vi "Test One Line State String Unwired.vi"(8 "error in (no error)":errorcluster) -> (0 "error out":errorcluster)   [LabVIEW 2013, in "JKI State Machine API - Tests.lvlib"]
uses:
  JKI State Machine API - Tests.lvlib
  source/JKI State Machine API.lvlib
  <vilib>/addons/_JKI Toolkits/Caraya/classes/Test/Test.lvclass
  <vilib>/addons/_JKI Toolkits/Caraya/classes/Assert/Assert.lvclass
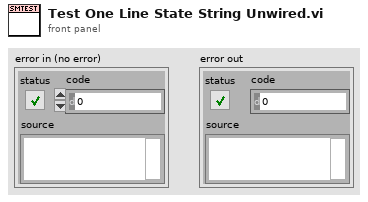
[diagram p1: front panel]
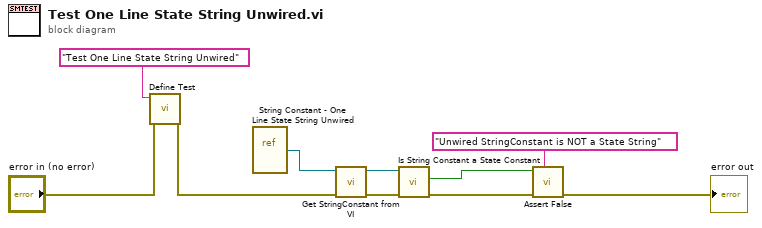
[diagram p0: block diagram]
diagram:
  n1 = call <vilib>:"Define Test.vi"("error in (no error)"="error in (no error)", "Label (VI Title)"="Test One Line State String Unwired") -> ("error out"=w9:errorcluster)  [unwired: 9 in]
  n2 = vi-ref "String Constant - One Line State String Unwired.vi"() -> (w6:refnum<vi>)
  n3 = call "Get StringConstant from VI.vi"("error in (no error)"=w9, "VI in"=w6) -> ("error out"=w5:errorcluster, "StringConstant out"=w4:refnum<vi>)  [unwired: 8 in]
  n4 = call "Is String Constant a State Constant.vi"("error in (no error)"=w5, "StrCnst Refnum"=w4) -> ("error out"=w7:errorcluster, "Is States Constant"=w10:bool)  [unwired: 7 in, 1 out]
  n5 = call <vilib>:"Assert False.vi"("Label"="Unwired StringConstant is NOT a State String", "error in (no error)"=w7, "False?"=w10) -> ("error out"=→"error out":errorcluster)  [unwired: 8 in]
